vi "Dashboard Main.vi"() -> ()   [LabVIEW 2013]
uses:
  AnnieFramework/DoubleSolenoidAction.ctl
  AnnieFramework/CollectorAction.ctl
  AnnieFramework/CollectorWrapAction.ctl
  AnnieFramework/CatchAction.ctl
  AnnieFramework/AutoStates.ctl
  AnnieFramework/RollerAction.ctl
  AnnieFramework/AutoMode.ctl
  AnnieFramework/PassState.ctl
  AnnieFramework/HotGoalDetectType.ctl
  AnnieFramework/LowGoalState.ctl
  <vilib>/sound2/lvsound2.llb/Sound Data Format.ctl
  TabEnum.ctl
  <vilib>/sound2/lvsound2.llb/Sampling Mode.ctl
  <vilib>/event_ctls.llb/eventvkey.ctl
  <vilib>/Rock Robotics/WPI/Dashboard/WPI_DashboardLogging Global.vi
  <vilib>/Utility/config.llb/Write Key (String).vi
  <vilib>/Utility/config.llb/Write Key (I32).vi
  <vilib>/sound2/lvsound2.llb/Sound Input Read (DBL).vi
  KariFramework/CheckImageDistance.vi
  <vilib>/Utility/config.llb/NI_LVConfig.lvlib
  <vilib>/Analysis/NI_AALPro.lvlib
panel:
  in  "Enable Vision":bool=TRUE
  out "Image Message":string="Timeout in Camera Communications"
  in  "Rec Mode":enum32{"Stop", "Record", "Playback"}(radio)
  in  "Dashboard Tab":T1(tab)
  in  "DisableKinect":bool=TRUE
  out "Version":string
  in  "XBox":bool
  in  "DisableLCD":bool=TRUE
  out "GroundPassState":T2
  in  "DisableRollerOut":bool=TRUE
  out "FrontSonar":dbl
  out "AtPressure":bool
  out "CatchState":T3
  out "CollectorWrapState":T4
  out "CollectorState":T5
  out "CollectorMotor":dbl
  out "ClapperState":T6
  out "RollerPneuState":T6
  out "FiringCylinder2":bool
  out "FiringCylinder1":bool
  out "Kicker":bool
  out "AutoDistanceDone?":bool
  out "BackSonar":dbl
  out "BottomLS":bool
  out "TopLS":bool
  in  "MaxMotorChange":dbl=1.5
  out "Error":bool
  out "Right Motor":dbl
  out "Left Motor":dbl
  in  "Camera Settings":T7={"Frame Rate"=30, "Compression"=30, "Size"=1} {"Frame Rate" scale=1.0..30.0; "Size" items=["640x480", "320x240", "160x120"]}
  out "Mode":T8(ring)=enum.""
  out "Camera IP":string="0.0.0.11"
  in  "DB Camera Config":bool
  out "fps":dbl format="%#.1g"
  out "Mbps":dbl format="%#.1g"
  out "Mbps 2":bool
  out "Pressure":i32
  out "RollerMotorState":T9
  in  "DisableServo":bool=TRUE
  out "ElevatedPassState":T2
  out "Arcade":bool
  out "TankDriveTime":dbl
  out "SonicShifter":bool
  out "StraightDrive":bool
  out "HalfDrive":bool
  out "ReverseDrive":bool
  out "LowGoalDumpState":T10
  out "KinectTriggered?":bool
  out "ServoAngle":dbl
  out "WebcamMatched? Copy":bool
  out "PitchDetected Copy":bool
  in  "PreScumbagWait":i32
  out "CheckGoalTime":u32
  in  "StartShootTime":i32=5000
  in  "DriveBackTime":i32=1000
  in  "DriveBackSpeed":dbl=-1.0
  in  "EndInLowGear?":bool=TRUE
  out "DriveElapsedTime":u32
  in  "AccelBackward":dbl=0.1
  in  "AccelForward":dbl=0.1
  in  "StartInLowGear?":bool=TRUE
  out "ShootTime":u32
  in  "BallSettleWait":i32=130
  in  "PreCheckGoalWait":i32=260
  in  "Slowdown":dbl=36.0
  in  "Brake":dbl=12.0
  in  "DriveDistance":dbl=36.0
  in  "DriveMinTime":i32=2000
  in  "DriveTimeout":i32=4000
  out "WasHot?":bool
  out "DriveTimeOut":bool
  out "CheckGoalTimedOut?":bool
  out "ElapsedTime":u32
  out "StateTime":u32
  out "CurrentState":T11
  out "RaiseArmTimedOut":bool
  out "LowerArmTimedOut":bool
  out "IDMatched?":bool
  in  "AutoID":i32=3061
  in  "AutoMode":T12=enum."OneBallCollector"
  in  "HotGoalType":T13
  in  "ResetSound?":bool
  out "Frequency":T14(graph)={"df"=0.0, "df"=2.205, "Power Spectrum (V^2 rms)"=array[5000 elements]}
  out "RawData":waveform(dbl)[](graph)=[{"t0"=timestamp(3478468008.2170343 s since 1904-01-01), "dt"=4.5351473922902495e-05, "Y"=array[10000 elements]}, {"t0"=timestamp(3478468008.2170343 s since 1904-01-01), "dt"=4.5351473922902495e-05, "Y"=array[10000 elements]}]
  out "MaxValue":dbl=1.242701184627817e-06 format="%#.5f"
  in  "Average":dbl=1.0
  in  "Freq Bandwidth":dbl=500.0 format="%#_13g"
  in  "Start Freq":dbl=4000.0 format="%#_13g"
  in  "SoundFormat":T15={"sample rate (S/s)"=22050.0, "number of channels"=2, "bits per sample"=16}
  in  "StopSoundDetect":bool
  in  "SoundCutoff":dbl=10.0 format="%#_13g"
  out "PitchDetected":bool
  in  "% Cutoff":dbl=0.5
  out "NumHot":i32
  out "NumProcessed":i32
  in  "NumSamples":i32=5
  out "ProcessImage?":bool
  in  "Finished?":bool
  in  "Hot?":bool
  in  "Score cutoff":dbl=0.5
  in  "Color System":u16(ring)=2 items=["RGB", "HSL", "HSV", "HSI"]
  out "Distance (ft)":dbl
  in  "Color Components":T16={"Hue"={112.0, 144.0}, "Sat"={202.0, 255.0}, "Val"={237.0, 255.0}} {"Val" scale=0.0..255.0; "Sat" scale=0.0..255.0; "Hue" scale=0.0..255.0 scale format="%#_3g"}
  out "LoopTime":u32=500
  in  "Calibrate?":bool
  in  "Reset?":bool
  in  "SaveCameraImage?":bool=TRUE
  in  "TestWebcam?":bool
  in  "RunWebcam?":bool
  out "WebcamImagesProcessed":i32
  in  "ResetWebcam?":bool
  in  "WebcamImages":i32=1
  in  "SaveWebcamImage?":bool
  out "WebcamMatched?":bool
  in  "WebcamStartTime (ms)":i32=2000
  in  "StopWebcam?":bool
  out "WebcamImage":T17(plugin-control)
  in  "height":i32=480
  in  "width":i32=640
  in  "driver":i32
  in  "Test Slider":dbl(slide) scale=0.0..100.0 scale format="%#_3g"
  in  "On/Off":bool caption="Solenoid"
  in  "Test Name":u16(ring) items=["Select the test to run...", "Example Test", "-------------------------------", "List of tests is built in robot code.", "Replace with your own automated tests."]
  in  "Test Tree":string(tree)
  in  "Motor":cluster{"Value":dbl, "Enable":bool} {"Value" scale=-1.0..1.0 scale format="%#_3g"}
  out "Progress":T18 {"Test Progress" scale=0.0..100.0}
  in  "Rev/Fwd":cluster{"Forward":bool, "Reverse":bool}
  in  "Test Ring":u16(ring) items=["Auto", "Fixed indoor", "Fixed outdoor 1", "Fixed outdoor 2", "Fixed fluorescent 1", "Fixed fluorescent 2", "Hold current"]
  in  "Listbox":i32(listbox)
  out "Tree":string(tree)
  out "ClosePressure":bool
  out "CloseDist":bool
  out "FarDist":bool
  out "Timer":u32
  in  "CountdownStartTime":u32=10
  in  "AutoLength":u32=10
  in  "TeleopLength":u32=140
  out "Status":T19(ring)
  in  "Beep?":bool=TRUE
  out "SoundFilePath":path
  out "Errors":T20(array[cluster])
  in  "Reset":bool
  out "Camera Image":T17(plugin-control)
  # "DRIVE"
  # "GENERAL"
  # "OUTPUT"
  # "CONFIG"
  # "DEPRECATED"
  # "COUNTDOWN"
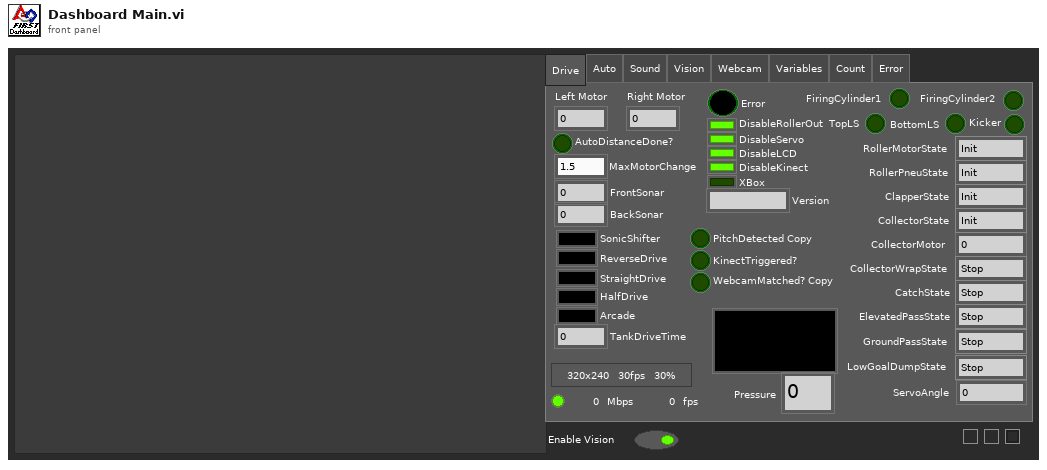
[diagram p1: front panel]
types:
  T1 = enum32{"Drive", "Auto", "Sound", "Vision", "Webcam", "Test", "Checklist", "Variables", "Count", "Error"}
  T2 = typedef "PassState.ctl" = enum16{"Stop", "Pass"}
  T3 = typedef "CatchAction.ctl" = enum16{"Stop", "PreCatch", "Catch"}
  T4 = typedef "CollectorWrapAction.ctl" = enum16{"Stop", "PreCollect", "Collect"}
  T5 = typedef "CollectorAction.ctl" = enum16{"Init", "Raise", "Lower", "Stop", "GetStatus"}
  T6 = typedef "DoubleSolenoidAction.ctl" = enum16{"Init", "Middle", "In", "Out"}
  T7 = cluster{"Frame Rate":i32, "Compression":i32, "Size":u16}
  T8 = enum8{"Tele-Op Disabled", "Tele-Op Enabled", "Auto Disabled", "Auto Enabled", "Test Disabled", "Test Enabled", ""}
  T9 = typedef "RollerAction.ctl" = enum16{"Init", "Off", "Forward", "Reverse"}
  T10 = typedef "LowGoalState.ctl" = enum16{"Stop", "Shoot"}
  T11 = typedef "AutoStates.ctl" = enum16{"Init", "LowerArmCheckGoal", "DriveBack", "Collect", "StopCollect", "LiftArm", "RaiseServo", "Drive", "ShootCollectorUp", "RaiseArm", "ShootCollectorDown", "Rotate1", "Rotate2", "Stop"}
  T12 = typedef "AutoMode.ctl" = enum16{"OneBallFront", "OneBallCollector", "TwoBallNormal", "TwoBallHot"}
  T13 = typedef "HotGoalDetectType.ctl" = enum16{"VisionTarget", "Kinect", "SoundDetect", "Webcam"}
  T14 = cluster{"df":dbl, "df":dbl, "Power Spectrum (V^2 rms)":dbl[]}
  T15 = typedef "Sound Data Format.ctl" = cluster{"sample rate (S/s)":dbl, "number of channels":i32, "bits per sample":i32}
  T16 = cluster{"Hue":cluster{dbl, dbl}, "Sat":cluster{dbl, dbl}, "Val":cluster{dbl, dbl}}
  T17 = typedef "IMAQ Image.ctl" = refnum<image>
  T18 = cluster{"Test Progress":u8, "Test Progress Text":string}
  T19 = enum8{"Disconnected", "E-Stop", "Disabled", "Enabled"}
  T20 = cluster{"status":bool, "code":i32, "location":string, "source":string}[]
  T21 = typedef "TabEnum.ctl" = enum32{"Drive", "Auto", "Sound", "Vision", "Webcam", "Variables", "Countdown", "Error"}
  T22 = typedef "Sampling Mode.ctl" = i32
  T23 = typedef "Image Type" = u32
  T24 = typedef "NI_LVConfig.lvlib/Config Data RefNum.ctl" = refnum<k1>
  T25 = typedef "Sound Input Task ID.ctl" = u32
  T26 = typedef "Sound Output Task ID.ctl" = u32
  T27 = cluster{"Digital Inputs":bool[], "Digital Outputs":bool[]}
  T28 = cluster{"Competition mode":bool, "Robot Link":bool, "Autonomous":bool, "Enabled":bool, "E-Stop":bool, "Simulated":bool, "TestMode":bool, "Docked Window":bool}
  T29 = typedef "CountdownAction.ctl" = enum16{"Start", "Reset", "Continue", "Idle"}
  T30 = cluster{"Boolean":bool, "Numeric":i32, "String":string, "String":string}[]
  T31 = cluster{cluster{dbl, dbl}, cluster{dbl, dbl}, cluster{dbl, dbl}}
  T32 = typedef "eventvkey.ctl" = enum16{"ASCII", "Enter", "Return", "Shift", "Ctrl", "Alt", "Cmd", "Opt", "Caps", "NumLock", "Clear", "Break", "Up", "Down", "Left", "Right", "Insert", "Delete", "Home", "End", "PageUp", "PageDown", "Escape", "Help", "Pause", "ScrollLock", "F1", "F2", "F3", "F4", "F5", "F6", "F7", "F8", "F9", "F10", "F11", "F12", "F13", "F14", "F15", "F16", "F17", "F18", "F19", "F20", "F21", "F22", "F23", "F24", "Play", "VolumeUp", "VolumeDown", "Mute", "Two Byte Char"}
  T33 = cluster{"Image Size":bool, "Image Type":bool, "Pixel Value":bool, "ROI Information":bool, "Zoom Factor":bool}
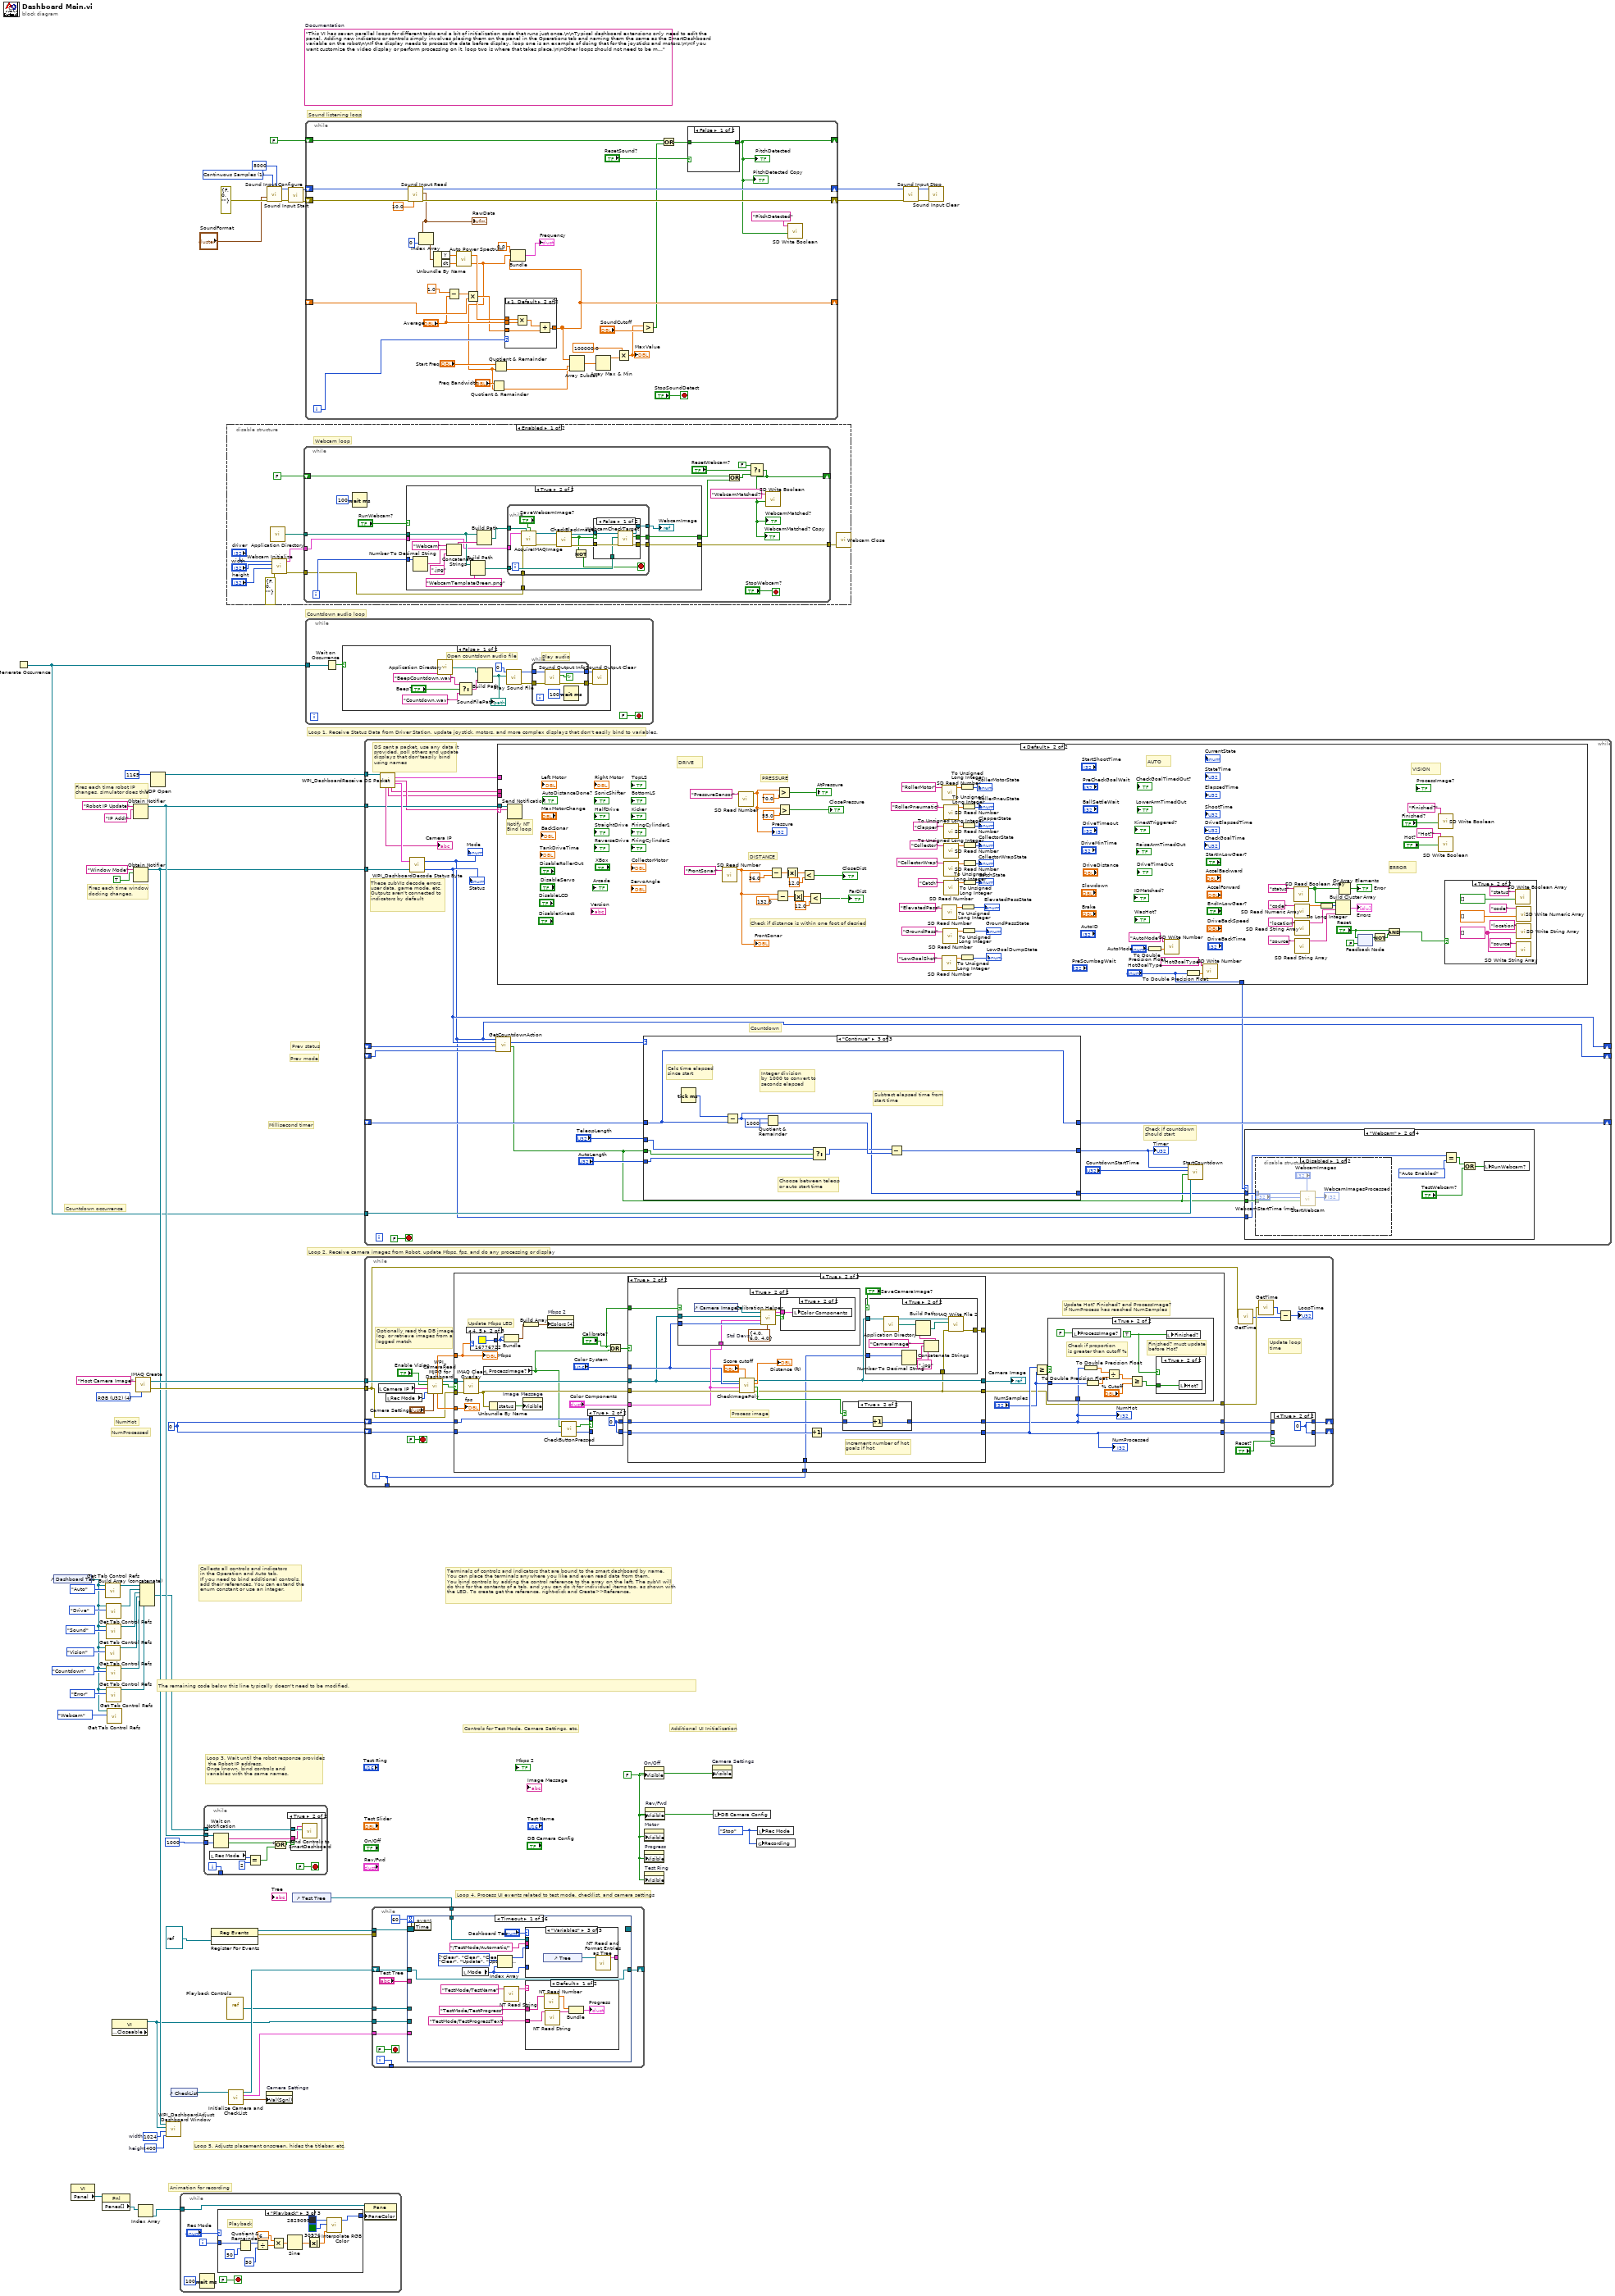
[diagram p0: block diagram]
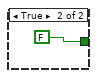
[diagram p2: hidden frame]
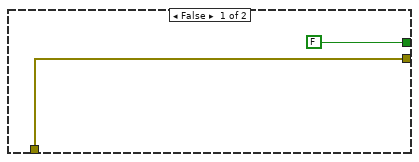
[diagram p4: hidden frame]
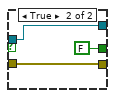
[diagram p5: hidden frame]
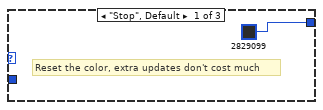
[diagram p8: hidden frame]
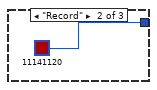
[diagram p9: hidden frame]
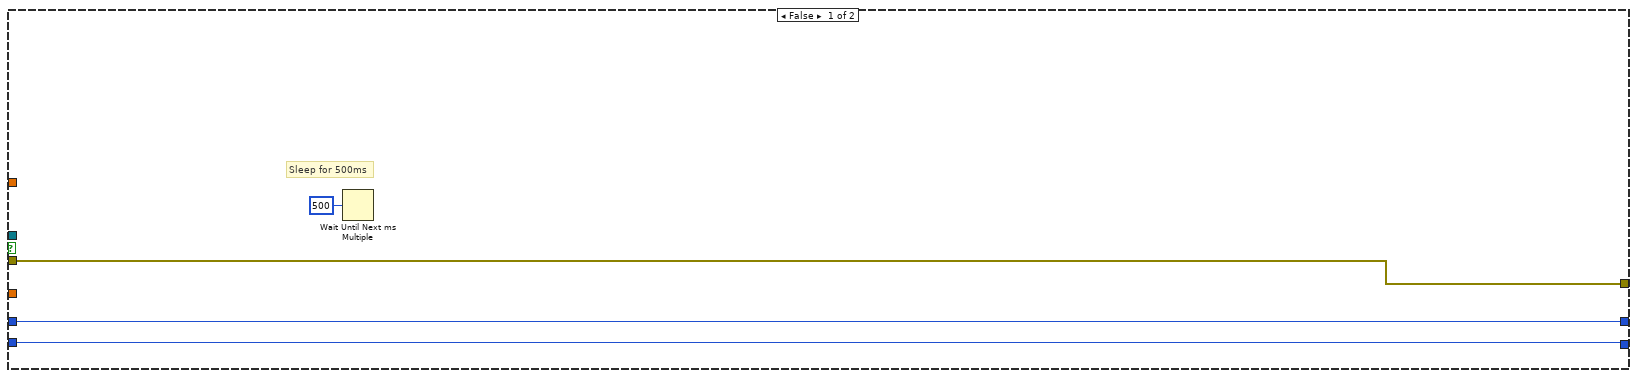
[diagram p12: hidden frame]
diagram:
  w23 = T22 1 items=["Finite Samples", "Continuous Samples"] ("sample mode")
  w26 = 0
  w32 = enum32{"Stop", "Record", "Playback"}."Stop" ("Rec Mode")
  w35 = 400  # height
  w36 = 1024  # width
  w49 = FALSE ("Visible")
  (unwired) "This VI has seven parallel loops for different tasks and a bit of initialization code that runs just once.\n\nTypical dashboard extensions only need to edit the panel. Adding new indicators or controls simply involves placing them on the panel in the Operations tab and naming them the same as the SmartDashboard variable on the robot\n\nIf the display needs to process the data before display, loop one is an example of doing that for the joysticks and motors.\n\nIf you want customize the video display or perform processing on it, loop two is where that takes place.\n\nOther loops should not need to be modified. They are pretty standard, and document the task they perform."  # Documentation
  w58 = T23 4 items=["Grayscale (U8)", "Grayscale (I16)", "Grayscale (SGL)", "Complex (CSG)", "RGB (U32)", "HSL (U32)", "RGB (U64)"] ("Image Type")
  # "Sound listening loop"
  # "Prev mode"
  # "Countdown audio loop"
  # "Countdown occurrence"
  # "Millisecond timer"
  # "Prev status"
  # "NumProcessed"
  # "NumHot"
  # "Controls for Test Mode, Camera Settings, etc."
  # "Additional UI Initialization"
  # "Animation for recording"
  # "Fires each time robot IP\nchanges, simulator does this"
  # "Fires each time window\ndocking changes."
  # "Collects all controls and indicators\nin the Operation and Auto tab.\nIf you need to bind additional controls,\nadd their references. You can extend the\nenum constant or use an integer."
  # "The remaining code below this line typically doesn't need to be modified."
  # "Loop 4. Process UI events related to test mode, checklist, and camera settings"
  # "Terminals of controls and indicators that are bound to the smart dashboard by name.\nYou can place the terminals anywhere you like and even read data from them.\nYou bind controls by adding the control reference to the array on the left. The subVI will\ndo this for the contents of a tab, and you can do it for individual items too, as shown with\nthe LED. To create get the reference, right-click and Create>>Reference."
  # "Loop 3. Wait until the robot response provides\n the Robot IP address.\nOnce known, bind controls and\nvariables with the same names."
  # "Loop 5. Adjusts placement onscreen, hides the titlebar, etc."
  # "Loop 1. Receive Status Data from Driver Station, update joystick, motors, and more complex displays that don't easily bind to variables."
  # "Loop 2. Receive camera images from Robot, update Mbps, fps, and do any processing or display"
  n1 = Generate Occurrence() -> (w25:refnum<k4>)
  n2 = control-ref of="Dashboard Tab"() -> (w2:refnum<vi>)
  n3 = property class="VI"() -> ("Panel"=w43:refnum<vi>)  [unwired: 2 in, 2 out]
  n4 = property class="Pnl"(reference=w43) -> ("Panes[]"=w44:refnum<vi>[])  [unwired: 1 in, 2 out]
  n5 = call <vilib>:"Get Tab Control Refs.vi"("Page Index"=TabEnum."Auto" ("Dashboard Tab"), "TabControl in"=w2) -> ("ControlsOnPage"=w30:refnum<vi>[])  [unwired: 9 in]
  n6 = call <vilib>:"Get Tab Control Refs.vi"("Page Index"=TabEnum."Vision" ("Dashboard Tab"), "TabControl in"=w2) -> ("ControlsOnPage"=w5:refnum<vi>[])  [unwired: 9 in]
  n7 = call <vilib>:"Get Tab Control Refs.vi"("Page Index"=TabEnum."Drive" ("Dashboard Tab"), "TabControl in"=w2) -> ("ControlsOnPage"=w27:refnum<vi>[])  [unwired: 9 in]
  n8 = call <vilib>:"Get Tab Control Refs.vi"("Page Index"=TabEnum."Sound" ("Dashboard Tab"), "TabControl in"=w2) -> ("ControlsOnPage"=w6:refnum<vi>[])  [unwired: 9 in]
  n9 = call <vilib>:"Get Tab Control Refs.vi"("Page Index"=TabEnum."Countdown" ("Dashboard Tab"), "TabControl in"=w2) -> ("ControlsOnPage"=w4:refnum<vi>[])  [unwired: 9 in]
  n10 = call <vilib>:"Get Tab Control Refs.vi"("Page Index"=TabEnum."Error" ("Dashboard Tab"), "TabControl in"=w2) -> ("ControlsOnPage"=w3:refnum<vi>[])  [unwired: 9 in]
  n11 = call <vilib>:"Get Tab Control Refs.vi"("Page Index"=TabEnum."Webcam" ("Dashboard Tab"), "TabControl in"=w2) -> ()  [unwired: 9 in, 1 out]
  n12 = property class="VI" props=["Front Panel.Closeable"]() -> (reference out=w31:refnum<vi>)  [unwired: 2 in, 2 out]
  n13 = Obtain Notifier(name (unnamed)="Robot IP Update", notification data type="IP Addr" ("name (unnamed)")) -> (notifier out=w52:refnum<notifier>)  [unwired: 2 in, 2 out]
  n14 = Obtain Notifier(name (unnamed)="Window Mode", notification data type=TRUE) -> (notifier out=w34:refnum<notifier>)  [unwired: 2 in, 2 out]
  n15 = call "IMAQ Create"("Image Name"="Host Camera Image", "Image Type"=w58) -> ("New Image"=w56:T17, "error out"=w55:errorcluster)  [unwired: 2 in, 1 out]
  n16 = Index Array(array=w44) -> (element=w42:refnum<vi>)  [unwired: 1 in]
  n17 = Build Array (concatenate)(w30, w27, w6, w5, w4, w3) -> (w29:refnum<vi>[])
  n18 = UDP Open(11:u16 1165 ("port")) -> (port=w59:refnum<k16>)  [unwired: 2 in, 4 out]
  n19 = call <vilib>:"WPI_DashboardAdjust Dashboard Window.vi"("height"=w35, "width"=w36, "reference in"=w31, "Notifier in"=w34) -> ()  [unwired: 8 in]
  n20 = control-ref of="CheckList"() -> (w33:refnum<vi>)
  n21 = while {
    tunnel: w42 -> [w62]
    i -> [w65]
    stop <- FALSE stop-if-true
    n22 = Wait (ms)(milliseconds to wait=u32 100) -> ()  [unwired: 1 out]
    n23 = case shown="\"Playback\"" "Rec Mode" {
      tunnel: w65 -> [_ _ w80]
      tunnel: [u32 2829099 ("Base Color") u32 11141120 ("Target Color") w69] -> w61
      frame "Stop", Default {
        # "Reset the color, extra updates don't cost much"
      }
      frame "Record" {
      }
      frame "Playback" {
        # "Playback"
        n24 = Quotient & Remainder(x=w80, y=u32 50 ("milliseconds to wait")) -> (x-y*floor(x/y)=w76:u32)  [unwired: 1 out]
        n25 = Divide(x=w76, y=u32 50 ("milliseconds to wait")) -> (x/y=w73:dbl)
        n26 = Multiply(x=6.283185307179586, y=w73) -> (x*y=w78:dbl)
        n27 = Sine(x=w78) -> (sin(x)=w77:dbl)
        n28 = Absolute Value(x=w77) -> (abs(x)=w70:dbl)
        n29 = call "Interpolate RGB Color.vi"("Proportion"=w70, "Target Color"=u32 30976, "Base Color"=u32 2829099) -> ("Result Color"=w69:u32)  [unwired: 8 in]
      }
    }
    n30 = property class="Pane"(reference=w62, "PaneColor"=w61) -> ()  [unwired: 1 in, 2 out]
  }
  n31 = while {
    tunnel: w29 -> [w91]
    tunnel: w52 -> [w89]
    tunnel: [w87] -> _
    tunnel: u32 1000 ("milliseconds to wait") -> [w86]
    i -> [w87]
    stop <- FALSE stop-if-true
    n32 = local read "Rec Mode"() -> (w82:enum32{"Stop", "Record", "Playback"})
    n33 = Wait on Notification(notifier=w89, timeout in ms (-1)=w86) -> (notification=w88:string, timed out?=w84:bool)  [unwired: 2 in, 2 out]
    n34 = Equal?(x=w82, y=u16 2 ("Rec Mode")) -> (x = y?=w83:bool)
    n35 = Compound Arithmetic op=OR(invert w84, w83) -> (w85:bool)
    n36 = case shown="True" w85 {
      tunnel: w91 -> [_ w93]
      tunnel: w88 -> [_ w92]
      frame False {
      }
      frame True {
        n37 = call <vilib>:"Bind Controls to SmartDashboard.vi"("Bound Control Refs"=w93, "Server IP Address"=w92) -> ()  [unwired: 10 in]
      }
    }
  }
  n38 = register-events(refnum<vi> refnum) -> (reference out=w40:refnum<event-registration>, error out=w39:errorcluster)  [unwired: 2 in]
  n39 = disable-structure shown="Enabled" {
    frame Enabled {
      # "Webcam loop"
      n40 = call <vilib>:"Application Directory.vi"() -> ("Application Directory"=w94:path)
      n41 = call "Webcam Initialize.vi"("error in"=errorcluster {"status"=FALSE, "code"=0, "source"=""}, "height (240)"="height", "width (320)"="width", "driver (0)"="driver") -> ("error out"=w97:errorcluster, "webcam image out"=w98:cluster{"image":u8[], "width":i32, "height":i32})  [unwired: 4 in, 1 out]
      n42 = while {
        tunnel: w94 -> [w117]
        tunnel: w98 -> [w115]
        tunnel: w97 -> [w114]
        tunnel: [w113] -> w96
        shift-right: [w103] -> _
        shift-left: FALSE -> [w109]
        i -> [w116]
        stop <- "StopWebcam?" stop-if-true
        n43 = Wait (ms)(milliseconds to wait=u32 100) -> ()  [unwired: 1 out]
        n44 = case shown="True" "RunWebcam?" {
          tunnel: [w118 w133] -> w113
          tunnel: [FALSE ("MatchFound?") w132] -> w108
          tunnel: w116 -> [_ w130]
          tunnel: w117 -> [_ w125]
          tunnel: w115 -> [_ w122]
          tunnel: w114 -> [w118 w121]
          frame False {
          }
          frame True {
            n45 = Number To Decimal String(number=w130) -> (decimal integer string=w129:string)  [unwired: 1 in]
            n46 = Concatenate Strings("Webcam", w129, ".jpg" ("string")) -> (w128:string)
            n47 = Build Path(base path=w125, name or relative path="WebcamTemplateGreen.png") -> (appended path=w124:path)
            n48 = Build Path(base path=w125, name or relative path=w128) -> (appended path=w127:path)
            n49 = while {
              tunnel: [w147] -> w133
              tunnel: [w146] -> w132
              tunnel: w127 -> [w145]
              tunnel: w124 -> [w143]
              tunnel: w122 -> [w136]
              tunnel: w121 -> [w135]
              tunnel: [w134] -> w120
              stop <- w137 stop-if-true
              n50 = call "AcquireIMAQImage.vi"("ImagePath"=w145, "SaveToDisk?"="SaveWebcamImage?", "error in"=w135, "webcam image in"=w136) -> ("error out"=w142:errorcluster, "ImageOut"=w140:T17)  [unwired: 6 in]
              n51 = call "CheckBlackImage.vi"("error in"=w142, "Image In"=w140) -> ("error out"=w141:errorcluster, "Black?"=w138:bool, "Image Out"=w139:T17)  [unwired: 7 in]
              n52 = Not(x=w138) -> (.not. x?=w137:bool)
              n53 = case shown="False" w138 {
                tunnel: w139 -> [w153 w154]
                tunnel: w141 -> [w152 w156]
                tunnel: [w151 w156] -> w147
                tunnel: [w150 FALSE ("MatchFound?")] -> w146
                tunnel: w143 -> [w149 _]
                tunnel: [w148 w154] -> w134
                frame False {
                  n54 = call "WebcamCheckTarget.vi"("error in"=w152, "TemplatePath"=w149, "ImageIn"=w153) -> ("error out"=w151:errorcluster, "MatchFound?"=w150:bool, "Image Out"=w148:T17)  [unwired: 6 in]
                }
                frame True {
                }
              }
            }
            "WebcamImage" <- w120
          }
        }
        n55 = Or(x=w109, y=w108) -> (x .or. y?=w106:bool)
        n56 = Select(t=FALSE, s="ResetWebcam?", f=w106) -> (s? t:f=w103:bool)
        "WebcamMatched?" <- w103
        "WebcamMatched? Copy" <- w103
        n57 = call <vilib>:"SD Write Boolean.vi"("Boolean"=w103, "Name"="WebcamMatched?") -> ()  [unwired: 8 in, 2 out]
      }
      n58 = call "Webcam Close.vi"("error in"=w96) -> ()  [unwired: 9 in, 1 out]
    }
    frame Disabled {
    }
  }
  n59 = vi-ref "Playback Controls.vi"() -> (w41:refnum<vi>)
  n60 = call "Initialize Camera and CheckList.vi"("ListBox in"=w33) -> ("Cluster"=w47:cluster{"value":i32, "value":i32, "index":i32}, "Array"=w48:cluster{string[]}[], "File Refnum"=w46:T24)  [unwired: 8 in]
  n61 = property on="Camera Settings" class="Clust (strict)"("Val(Sgnl)"=w47) -> ()  [unwired: 2 in, 2 out]
  n62 = call <vilib>:"Sound Input Configure.vi"("number of samples/ch"=8000, "sample mode"=w23, "error in (no error)"=errorcluster {"status"=FALSE, "code"=0, "source"=""}, "sound format"="SoundFormat") -> ("error out"=w20:errorcluster, "task ID"=w21:T25)  [unwired: 6 in]
  n63 = call <vilib>:"Sound Input Start.vi"("error in (no error)"=w20, "task ID"=w21) -> ("error out"=w19:errorcluster, "task ID out"=w18:T25)  [unwired: 8 in]
  n64 = control-ref of="Test Tree"() -> (w45:refnum<vi>)
  n65 = while {
    shift-right: [w189] -> w17
    shift-left: w19 -> [w191]
    shift-right: [w190] -> w16
    shift-left: w18 -> [w192]
    shift-right: [w186] -> _
    shift-left: _ -> [w188]
    shift-right: [w157] -> _
    shift-left: FALSE -> [w162]
    i -> [w187]
    stop <- "StopSoundDetect" stop-if-true
    n66 = call-poly <vilib>:"Sound Input Read.vi"("timeout (sec)"=10.0, "error in (no error)"=w191, "task ID"=w192) -> ("error out"=w189:errorcluster, "data"=w184:waveform(dbl)[], "task ID out"=w190:T25)  [unwired: 6 in]
    "RawData" <- w184
    n67 = Index Array(array=w184, index=0) -> (element=w180:waveform(dbl))
    n68 = Unbundle By Name(w180) -> ("Y"=w181:dbl[], "dt"=w178:dbl)
    n69 = Subtract(x=1.0, y="Average") -> (x-y=w174:dbl)
    n70 = call <vilib>:"Auto Power Spectrum.vi"("dt"=w178, "Signal (V)"=w181) -> ("df"=w170:dbl, "Power Spectrum (V^2 rms)"=w177:dbl[])
    n71 = Multiply(x=w174, y=w188) -> (x*y=w173:dbl[])
    n72 = Quotient & Remainder(x="Freq Bandwidth", y=w170) -> (floor(x/y)=w168:dbl)  [unwired: 1 out]
    n73 = Quotient & Remainder(x="Start Freq", y=w170) -> (floor(x/y)=w169:dbl)  [unwired: 1 out]
    n74 = case shown="1, Default" w187 {
      tunnel: w177 -> [w196 w201]
      tunnel: "Average" -> [_ w200]
      tunnel: w173 -> [_ w198]
      tunnel: [w196 w197] -> w186
      frame 0 {
      }
      frame 1, Default {
        n75 = Multiply(x=w201, y=w200) -> (x*y=w199:dbl[])
        n76 = Add(x=w199, y=w198) -> (x+y=w197:dbl[])
      }
    }
    n77 = Bundle("df"=0.0, "df"=w170, "Power Spectrum (V^2 rms)"=w186) -> (→"Frequency":T14)  [unwired: 1 in]
    n78 = Array Subset(array=w186, index=w169, length=w168) -> (w167:dbl[])
    n79 = Array Max & Min(array=w167) -> (max value=w166:dbl)  [unwired: 3 out]
    n80 = Multiply(x=100000.0, y=w166) -> (x*y=w163:dbl)
    "MaxValue" <- w163
    n81 = Greater?(x=w163, y="SoundCutoff") -> (0:w161:bool)
    n82 = Or(x=w162, y=w161) -> (x .or. y?=w160:bool)
    n83 = case shown="False" "ResetSound?" {
      tunnel: w160 -> [w194 _]
      tunnel: [w194 FALSE] -> w157
      frame False {
      }
      frame True {
      }
    }
    "PitchDetected" <- w157
    "PitchDetected Copy" <- w157
    n84 = call <vilib>:"SD Write Boolean.vi"("Boolean"=w157, "Name"="PitchDetected") -> ()  [unwired: 8 in, 2 out]
  }
  n85 = while {
    tunnel: w25 -> [w202]
    stop <- FALSE stop-if-true
    n86 = Wait on Occurrence(2:w202) -> (0:w204:bool)  [unwired: 2 in]
    n87 = case shown="False" w204 {
      frame False {
        # "Play audio"
        # "Open countdown audio file"
        n88 = call <vilib>:"Application Directory.vi"() -> ("Application Directory"=w205:path)
        n89 = Select(t="BeepCountdown.wav" ("name or relative path"), s="Beep?", f="Countdown.wav" ("name or relative path")) -> (s? t:f=w207:string)
        n90 = Build Path(base path=w205, name or relative path=w207) -> (appended path=w206:path)
        "SoundFilePath" <- w206
        n91 = call <vilib>:"Play Sound File.vi"("path"=w206, "device ID"=u32 0) -> ("error out"=w214:errorcluster, "task ID"=w213:T26)  [unwired: 8 in]
        n92 = while {
          tunnel: w214 -> [w216]
          tunnel: w213 -> [w220]
          tunnel: [w219] -> w212
          tunnel: [w217] -> w211
          stop <- w218 continue-if-true
          n93 = call <vilib>:"Sound Output Info.vi"("error in (no error)"=w216, "task ID"=w220) -> ("error out"=w217:errorcluster, "is playing?"=w218:bool, "task ID out"=w219:T26)  [unwired: 6 in, 1 out]
          n94 = Wait (ms)(milliseconds to wait=u32 100) -> ()  [unwired: 1 out]
        }
        n95 = call <vilib>:"Sound Output Clear.vi"("error in (no error)"=w211, "task ID"=w212) -> ()  [unwired: 9 in, 1 out]
      }
      frame True {
      }
    }
  }
  n96 = while {
    tunnel: w59 -> [w244]
    tunnel: w52 -> [w241]
    tunnel: w34 -> [w243]
    shift-right: [w236] -> _
    shift-left: _ -> [w235]
    shift-right: [w233] -> _
    shift-left: _ -> [w232]
    tunnel: w25 -> [w227]
    shift-right: [w222] -> _
    shift-left: _ -> [w224]
    stop <- FALSE stop-if-true
    # "Check if countdown\nshould start"
    # "Countdown"
    # "DS sent a packet. use any data it\nprovided, poll others and update\ndisplays that don'teasily bind\nusing names"
    # "These subVIs decode errors, user data, game mode, etc.\nOutputs aren't connected to indicators by default"
    n97 = call <vilib>:"WPI_DashboardReceive DS Packet.vi"("Recv Socket"=w244) -> ("Driver Station"=w237:T27, "Robot IP Address"=w240:string, "Status"=w245:T28, "Camera IP Address"=→"Camera IP":string, "Low Priority User Data"=w239:string, "High Priority User Data"=w238:string)  [unwired: 1 in, 8 out]
    n98 = call <vilib>:"WPI_DashboardDecode Status Byte.vi"("Window Mode Notifier"=w243, "Status"=w245) -> ("Status"=w236:T19, "Mode"=w222:T8)
    "Mode" <- w222
    "Status" <- w236
    n99 = call "GetCountdownAction.vi"("PrevMode"=w224, "PrevStatus"=w235, "CurrentStatus"=w236, "CurrentMode"=w222) -> ("Teleop?"=w225:bool, "Action"=w234:T29)  [unwired: 6 in]
    n100 = case shown="Default" w240 {
      selector: w240 -> [_ w349]
      tunnel: w241 -> [_ w350]
      tunnel: w239 -> [_ _]
      tunnel: w238 -> [_ _]
      tunnel: w237 -> [_ _]
      tunnel: [_ "HotGoalType"] -> w223
      frame "0.0.0.0" {
        # "DS not sending packets, or no robot exists yet.\nDon't poll the variables"
      }
      frame Default {
        # "Check if distance is within one foot of desried"
        # "ERROR"
        # "DISTANCE"
        # "PRESSURE"
        # "VISION"
        # "AUTO"
        # "DRIVE"
        # "Notify NT\nBind loop"
        n101 = Send Notification(notification=w349, notifier=w350) -> ()  [unwired: 1 in, 2 out]
        n102 = call <vilib>:"SD Read Number.vi"("Name"="FrontSonar") -> ("Numeric"=w300:dbl)  [unwired: 8 in, 2 out]
        "FrontSonar" <- w300
        n103 = call <vilib>:"SD Read Number.vi"("Name"="PressureSensor") -> ("Numeric"=w299:dbl)  [unwired: 8 in, 2 out]
        "Pressure" <- w299
        n104 = Subtract(x=w300, y=36.0) -> (x-y=w307:dbl)
        n105 = Subtract(x=w300, y=132.0) -> (x-y=w302:dbl)
        n106 = Greater?(x=w299, y=70.0) -> (0:→"AtPressure":bool)
        n107 = Greater?(x=w299, y=55.0) -> (0:→"ClosePressure":bool)
        n108 = Absolute Value(x=w307) -> (abs(x)=w306:dbl)
        n109 = Absolute Value(x=w302) -> (abs(x)=w303:dbl)
        n110 = Less?(x=w306, y=12.0) -> (x < y?=→"CloseDist":bool)
        n111 = Less?(x=w303, y=12.0) -> (x < y?=→"FarDist":bool)
        n112 = call <vilib>:"SD Read Number.vi"("Name"="LowGoalShot") -> ("Numeric"=w283:dbl)  [unwired: 8 in, 2 out]
        n113 = call <vilib>:"SD Read Number.vi"("Name"="RollerMotor") -> ("Numeric"=w297:dbl)  [unwired: 8 in, 2 out]
        n114 = call <vilib>:"SD Read Number.vi"("Name"="ElevatedPass") -> ("Numeric"=w291:dbl)  [unwired: 8 in, 2 out]
        n115 = call <vilib>:"SD Read Number.vi"("Name"="GroundPass") -> ("Numeric"=w290:dbl)  [unwired: 8 in, 2 out]
        n116 = call <vilib>:"SD Read Number.vi"("Name"="RollerPneumatic") -> ("Numeric"=w327:dbl)  [unwired: 8 in, 2 out]
        n117 = call <vilib>:"SD Read Number.vi"("Name"="Clapper") -> ("Numeric"=w325:dbl)  [unwired: 8 in, 2 out]
        n118 = call <vilib>:"SD Read Number.vi"("Name"="Collector") -> ("Numeric"=w322:dbl)  [unwired: 8 in, 2 out]
        n119 = call <vilib>:"SD Read Number.vi"("Name"="CollectorWrap") -> ("Numeric"=w319:dbl)  [unwired: 8 in, 2 out]
        n120 = call <vilib>:"SD Read Number.vi"("Name"="Catch") -> ("Numeric"=w316:dbl)  [unwired: 8 in, 2 out]
        n121 = To Unsigned Long Integer(number=w297) -> (unsigned 32bit integer=→"RollerMotorState":u32)
        n122 = To Unsigned Long Integer(number=w283) -> (unsigned 32bit integer=→"LowGoalDumpState":u32)
        n123 = To Unsigned Long Integer(number=w291) -> (unsigned 32bit integer=→"ElevatedPassState":u32)
        n124 = To Unsigned Long Integer(number=w327) -> (unsigned 32bit integer=→"RollerPneuState":u32)
        n125 = To Unsigned Long Integer(number=w325) -> (unsigned 32bit integer=→"ClapperState":u32)
        n126 = To Unsigned Long Integer(number=w290) -> (unsigned 32bit integer=→"GroundPassState":u32)
        n127 = To Unsigned Long Integer(number=w322) -> (unsigned 32bit integer=→"CollectorState":u32)
        n128 = To Unsigned Long Integer(number=w319) -> (unsigned 32bit integer=→"CollectorWrapState":u32)
        n129 = To Unsigned Long Integer(number=w316) -> (unsigned 32bit integer=→"CatchState":u32)
        n130 = To Double Precision Float(number="AutoMode") -> (double precision float=w293:dbl)
        n131 = call <vilib>:"SD Write Number.vi"("Numeric"=w293, "Name"="AutoMode") -> ()  [unwired: 8 in, 2 out]
        n132 = To Double Precision Float(number="HotGoalType") -> (double precision float=w286:dbl)
        n133 = call <vilib>:"SD Write Number.vi"("Numeric"=w286, "Name"="HotGoalType") -> ()  [unwired: 8 in, 2 out]
        n134 = call <vilib>:"SD Read Boolean Array.vi"("Name"="status") -> ("Boolean Array"=w338:bool[])  [unwired: 8 in, 2 out]
        n135 = call <vilib>:"SD Read Numeric Array.vi"("Name"="code") -> ("Numeric Array"=w337:dbl[])  [unwired: 8 in, 2 out]
        n136 = call <vilib>:"SD Read String Array.vi"("Name"="location") -> ("String Array"=w336:string[])  [unwired: 9 in, 1 out]
        n137 = call <vilib>:"SD Read String Array.vi"("Name"="source") -> ("String Array"=w335:string[])  [unwired: 9 in, 1 out]
        n138 = To Long Integer(number=w337) -> (32bit integer=w343:i32[])
        n139 = Build Cluster Array(w338, w343, w336, w335) -> (→"Errors":T30)
        n140 = Or Array Elements(Boolean array=w338) -> (logical OR=→"Error":bool)
        n141 = feedback #1(FALSE ("Reset")) -> (w346:bool)
        n142 = feedback-in #1("Reset") -> ()
        n143 = Not(x=w346) -> (.not. x?=w345:bool)
        n144 = And(x="Reset", y=w345) -> (x .and. y?=w344:bool)
        n145 = call <vilib>:"SD Write Boolean.vi"("Boolean"="Finished?", "Name"="Finished?") -> ()  [unwired: 8 in, 2 out]
        n146 = call <vilib>:"SD Write Boolean.vi"("Boolean"="Hot?", "Name"="Hot?") -> ()  [unwired: 8 in, 2 out]
        n147 = case shown="True" w344 {
          frame False {
          }
          frame True {
            w351 = string[] [] ("String Array")
            n148 = call <vilib>:"SD Write Boolean Array.vi"("Boolean Array"=bool[] [], "Name"="status") -> ()  [unwired: 8 in, 2 out]
            n149 = call <vilib>:"SD Write Numeric Array.vi"("Numeric Array"=dbl[] [], "Name"="code") -> ()  [unwired: 8 in, 2 out]
            n150 = call <vilib>:"SD Write String Array.vi"("String Array"=w351, "Name"="location") -> ()  [unwired: 8 in, 2 out]
            n151 = call <vilib>:"SD Write String Array.vi"("String Array"=w351, "Name"="source") -> ()  [unwired: 8 in, 2 out]
          }
        }
      }
    }
    n152 = case shown="\"Continue\"" w234 {
      tunnel: "TeleopLength" -> [w262 _ w275]
      tunnel: "AutoLength" -> [w261 _ w274]
      tunnel: [w265 w266 w273] -> w229
      tunnel: [w264 w267 w272] -> w233
      tunnel: w232 -> [_ w267 w272]
      tunnel: w225 -> [w263 _ w276]
      tunnel: [u32 0 ("millisecond timer value") w266 w268] -> w226
      frame "Start", Default {
        # "Choose between auto and teleop start times"
        n153 = Select(t=w262, s=w263, f=w261) -> (s? t:f=w265:u32)
        n154 = Tick Count (ms)() -> (millisecond timer value=w264:u32)
      }
      frame "Reset", "Idle" {
        w266 = u32 0 ("AutoStartTime")
      }
      frame "Continue" {
        # "Subtract elapsed time from\nstart time"
        # "Choose between teleop\nor auto start time"
        # "Integer division\nby 1000 to convert to\nseconds elapsed"
        # "Calc time elapsed\nsince start"
        n155 = Tick Count (ms)() -> (millisecond timer value=w269:u32)
        n156 = Subtract(x=w269, y=w272) -> (x-y=w268:u32)
        n157 = Quotient & Remainder(x=w268, y=u32 1000) -> (floor(x/y)=w271:u32)  [unwired: 1 out]
        n158 = Select(t=w275, s=w276, f=w274) -> (s? t:f=w270:u32)
        n159 = Subtract(x=w270, y=w271) -> (x-y=w273:u32)
      }
    }
    "Timer" <- w229
    n160 = call "StartCountdown.vi"("CountdownOccurrence"=w227, "Teleop?"=w225, "CountdownStartTime"="CountdownStartTime", "Time"=w229) -> ()  [unwired: 8 in]
    n161 = case shown="\"Webcam\"" w223 {
      tunnel: w226 -> [_ w253 _ _]
      tunnel: w225 -> [_ w252 _ _]
      tunnel: w222 -> [_ w251 _ _]
      frame "VisionTarget", Default {
      }
      frame "Webcam" {
        n162 = disable-structure shown="Disabled" {
          disable-tunnel: w253 -> [w259 _]
          disable-tunnel: w252 -> [w258 _]
          frame Disabled {
            n163 = call "StartWebcam.vi"("NumWebcamImages"="WebcamImages", "Teleop?"=w258, "WebcamStartTime (ms)"="WebcamStartTime (ms)", "ElapsedTime (ms)"=w259) -> ("WebcamImagesProcessed"=→"WebcamImagesProcessed":i32, "ResetWebcam?"=w255:bool)  [unwired: 6 in]
          }
          frame Enabled {
          }
        }
        n164 = Equal?(x=w251, y=T8."Auto Enabled") -> (x = y?=w249:bool)
        n165 = Or(x=w249, y="TestWebcam?") -> (x .or. y?=w247:bool)
        n166 = local write "RunWebcam?"(w247) -> ()
      }
      frame "Kinect" {
      }
      frame "SoundDetect" {
      }
    }
  }
  n167 = while {
    tunnel: w56 -> [w379]
    tunnel: w55 -> [w364]
    tunnel: [w358] -> _
    shift-right: [w359] -> _
    shift-left: w26 -> [w369]
    shift-right: [w360] -> _
    shift-left: w26 -> [w370]
    i -> [w358]
    stop <- FALSE stop-if-true
    # "Update loop\ntime"
    # "Optionally read the DB image,\nlog, or retrieve images from a\nlogged match"
    n168 = local read "Camera IP"() -> (w372:string)
    n169 = local read "Rec Mode"() -> (w371:enum32{"Stop", "Record", "Playback"})
    n170 = call <vilib>:"WPI_CameraRead MJPG for Dashboard.vi"("Camera Settings"="Camera Settings", "Rec Mode"=w371, "Camera IP"=w372, "Enable"="Enable Vision", "Refnum in"=w379) -> ("Active"=w376:bool, "Refnum out"=w378:T17, "FPS"=w375:dbl, "Bandwidth (Mbps)"=w374:dbl)  [unwired: 3 in]
    n171 = case shown="True" w376 {
      tunnel: w378 -> [_ w410]
      tunnel: w374 -> [_ w409]
      tunnel: w375 -> [_ w408]
      tunnel: w370 -> [w385 w398]
      tunnel: w369 -> [w386 w397]
      tunnel: [w386 w403] -> w362
      tunnel: [w385 w402] -> w361
      tunnel: [w384 w400] -> w367
      tunnel: w364 -> [w384 w399]
      tunnel: w358 -> [_ w388]
      frame False {
        # "Sleep for 500ms"
        n172 = Wait Until Next ms Multiple(millisecond multiple=u32 500) -> ()  [unwired: 1 out]
      }
      frame True {
        # "Update Hot? Finished? and ProcessImage?\nIf NumProcess has reached NumSamples"
        # "Update Mbps LED"
        n173 = call "IMAQ Clear Overlay"("error in (no error)"=w399, "Image"=w410) -> ("error out"=w405:errorcluster, "Image Out"=w407:T17)  [unwired: 1 in, 7 out]
        n174 = case shown="4, 5" w409 {
          tunnel: [u32 6618880 ("Color Box") u32 16776722 ("Color Box") u32 16716800 ("Color Box")] -> w411
          frame Default {
          }
          frame 4, 5 {
          }
          frame 6.. {
          }
        }
        n175 = local read "ProcessImage?"() -> (w390:bool)
        n176 = Unbundle By Name(w405) -> ("status"=w414:bool)
        n177 = Bundle("Color Box"=w411, "Color Box"=w411) -> (w413:cluster{"Color Box":u32, "Color Box":u32})  [unwired: 1 out]
        n178 = property on="Image Message" class="Str"("Visible"=w414) -> ()  [unwired: 2 in, 2 out]
        n179 = Build Array(w413) -> (w412:cluster{"Color Box":u32, "Color Box":u32}[])
        n180 = property on="Mbps 2" class="Bool (strict)"("Colors [4]"=w412) -> ()  [unwired: 2 in, 2 out]
        n181 = call "CheckButtonPressed.vi"("Button"=w390) -> ("Pressed?"=w394:bool)  [unwired: 9 in, 1 out]
        n182 = case shown="True" w394 {
          tunnel: w398 -> [w416 _]
          tunnel: w397 -> [w415 _]
          tunnel: [w416 w417] -> w396
          tunnel: [w415 w417] -> w395
          frame False {
          }
          frame True {
            w417 = 0
          }
        }
        n183 = Or(x="Calibrate?", y=w390) -> (x .or. y?=w391:bool)
        n184 = case shown="True" w391 {
          tunnel: w407 -> [w428 w438]
          tunnel: [w428 w435] -> w406
          tunnel: w396 -> [w430 w444]
          tunnel: w395 -> [w431 w446]
          tunnel: w405 -> [w429 w447]
          tunnel: [w429 w434] -> w400
          tunnel: [w431 w445] -> w403
          tunnel: [w430 w443] -> w402
          tunnel: "Color Components" -> [_ w440]
          tunnel: "Color System" -> [_ w439]
          tunnel: "Calibrate?" -> [_ w437]
          tunnel: [_ w433] -> _
          tunnel: w388 -> [_ w432]
          frame False {
          }
          frame True {
            # "Process image"
            # "Increment number of hot\ngoals if hot"
            n185 = case shown="True" w437 {
              tunnel: w439 -> [_ w464]
              tunnel: w440 -> [_ w463]
              tunnel: w438 -> [_ w462]
              frame False {
              }
              frame True {
                w465 = cluster{"Hue":dbl, "Sat":dbl, "Val":dbl} {"Hue"=4.0, "Sat"=6.0, "Val"=4.0}  # Std Devs
                n186 = control-ref of="Camera Image"() -> (w461:refnum<vi>)
                n187 = call "Calibration Helper.vi"("Std Devs"=w465, "Color Mode"=w464, "Color Components"=w463, "Image"=w462, "Image Ctl Refnum"=w461) -> ("Changed"=w459:bool, "output color"=w460:T31)  [unwired: 5 in]
                n188 = case shown="True" w459 {
                  tunnel: w460 -> [_ w466]
                  frame False {
                  }
                  frame True {
                    n189 = local write "Color Components"(w466) -> ()
                  }
                }
              }
            }
            n190 = call-poly "CheckImagePoly.vi"("Score cutoff"="Score cutoff", "error in"=w447, "Color Components"=w440, "Color System"=w439, "Image"=w438) -> ("error out"=w434:errorcluster, "Hot?"=w441:bool, "Distance (ft)"=→"Distance (ft)":dbl, "Image out"=w435:T17)  [unwired: 3 in]
            n191 = Increment(x=w446) -> (x+1=w445:i32)
            n192 = case shown="True" w441 {
              tunnel: w444 -> [w467 w469]
              tunnel: [w467 w468] -> w443
              frame False {
              }
              frame True {
                n193 = Increment(x=w469) -> (x+1=w468:i32)
              }
            }
            n194 = case shown="True" "SaveCameraImage?" {
              tunnel: w435 -> [_ w458]
              tunnel: w434 -> [_ w457]
              tunnel: [_ w456] -> w433
              tunnel: w432 -> [_ w453]
              frame False {
              }
              frame True {
                n195 = call <vilib>:"Application Directory.vi"() -> ("Application Directory"=w449:path)
                n196 = Number To Decimal String(number=w453) -> (decimal integer string=w452:string)  [unwired: 1 in]
                n197 = Concatenate Strings("CameraImage", w452, ".jpg" ("string")) -> (w450:string)
                n198 = Build Path(base path=w449, name or relative path=w450) -> (appended path=w455:path)
                n199 = call-poly "IMAQ Write File 2"("error in (no error)"=w457, "File Path"=w455, "Image"=w458) -> ("error out"=w456:errorcluster)  [unwired: 7 in, 1 out]
              }
            }
          }
        }
        "Camera Image" <- w406
        "NumHot" <- w402
        "NumProcessed" <- w403
        n200 = Greater Or Equal?(x=w403, y="NumSamples") -> (x >= y?=w404:bool)
        n201 = case shown="True" w404 {
          tunnel: w402 -> [_ w425]
          tunnel: "NumSamples" -> [_ w426]
          frame False {
          }
          frame True {
            w418 = TRUE ("Finished?")
            # "Finished? must update\nbefore Hot?"
            # "Check if proportion\nis greater than cutoff %"
            n202 = local write "ProcessImage?"(FALSE ("ProcessImage?")) -> ()
            n203 = To Double Precision Float(number=w425) -> (double precision float=w423:dbl)
            n204 = To Double Precision Float(number=w426) -> (double precision float=w424:dbl)
            n205 = Divide(x=w423, y=w424) -> (x/y=w422:dbl)
            n206 = Greater Or Equal?(x=w422, y="% Cutoff") -> (x >= y?=w420:bool)
            n207 = case shown="True" w418 {
              tunnel: w420 -> [_ w427]
              frame False {
              }
              frame True {
                n208 = local write "Hot?"(w427) -> ()
              }
            }
            n209 = local write "Finished?"(w418) -> ()
          }
        }
        "Mbps" <- w409
        "fps" <- w408
      }
    }
    n210 = call "GetTime.vi"("error in"=w364) -> ("Time"=w366:u32)
    n211 = call "GetTime.vi"("error in"=w367) -> ("Time"=w368:u32)
    n212 = case shown="True" "Reset?" {
      tunnel: w362 -> [w381 _]
      tunnel: w361 -> [w382 _]
      tunnel: [w382 w383] -> w360
      tunnel: [w381 w383] -> w359
      frame False {
      }
      frame True {
        w383 = 0
      }
    }
    n213 = Subtract(x=w368, y=w366) -> (x-y=→"LoopTime":u32)
  }
  n214 = while {
    tunnel: w48 -> [w480]
    shift-right: [w479] -> _
    shift-left: w46 -> [w478]
    tunnel: [w477] -> _
    tunnel: w45 -> [w476]
    tunnel: w41 -> [w475]
    tunnel: w40 -> [w474]
    tunnel: w39 -> [_]
    tunnel: w31 -> [w473]
    i -> [w477]
    stop <- FALSE stop-if-true
    n215 = event shown="[0] Timeout" {
      selector: w474 -> [_ _ _ _ _ _ _ _ _ _ _ _ _ _ _ _]
      dyn-events: [_ _ _ _ _ _ _ _ _ _ _ _ _ w718 _ _] -> _
      timeout: u32 60 ("milliseconds to wait") -> [_ _ _ _ _ _ _ _ _ _ _ _ _ _ _ _]
      tunnel: w476 -> [w490 _ _ _ _ _ _ _ _ _ _ _ _ _ _ _]
      tunnel: "Test Tree" -> [_ _ _ _ _ _ _ _ w687 w695 w697 w701 w709 _ _ _]
      tunnel: w480 -> [_ w514 _ _ _ _ w651 w681 _ _ _ _ _ _ _ _]
      tunnel: [w484 w513 w612 w617 w625 w637 w650 w674 w686 w693 w696 w700 w708 w720 w734 w735] -> w479
      tunnel: w478 -> [w484 w513 w612 w617 w625 w637 w649 w674 w686 w693 w696 w700 w708 w720 w734 w735]
      tunnel: w475 -> [_ _ _ _ _ _ _ _ _ _ _ _ _ w721 _ w738]
      tunnel: w473 -> [_ _ _ _ _ _ _ _ _ _ _ _ _ w716 _ _]
      event Timeout {
        w489 = enum16{"Update", "Clear"}[] [enum."Clear", enum."Clear", enum."Clear", enum."Clear", enum."Update", enum."Update", enum."Clear"] items=["Update", "Clear"]
        n216 = event-data() -> ()  [unwired: 1 in, 1 out]
        n217 = local read "Mode"() -> (w487:T8)
        n218 = Index Array(array=w489, index=w487) -> (element=w488:enum16{"Update", "Clear"})
        n219 = call <vilib>:"NT Read String.vi"("Name"="TestMode/TestName") -> ("String"=w493:string)  [unwired: 9 in, 1 out]
        n220 = case shown="\"Variables\"" "Dashboard Tab" {
          tunnel: w490 -> [_ w503 _]
          tunnel: "/TestMode/Automatic/" ("Name Pattern") -> [_ w502 _]
          tunnel: w488 -> [_ w501 _]
          tunnel: w487 -> [_ w499 _]
          tunnel: [_ _ w505] -> _
          frame "Auto", Default {
          }
          frame "Test" {
            w498 = -2 ("Active Item:Row Number")
            n221 = call <vilib>:"NT Read and Format Entries as Tree.vi"("Operation"=w501, "Name Pattern"=w502, "Tree Refnum"=w503) -> ()  [unwired: 7 in, 2 out]
            n222 = Index Array(array=u32[] [14013909, 14013909, 14013909, 14013909, 14013909, 16777215, 14013909], index=w499) -> (element=w497:u32)
            n223 = property on="Test Tree" class="Tree (strict)"("Active Item Row Number"=w498, "ActiveColNum"=w498, "CellBG"=w497, "Active Item Row Number"=-1 ("Active Item:Row Number"), "CellBG"=u32 5789784 ("Color Box")) -> ()  [unwired: 2 in, 2 out]
          }
          frame "Variables" {
            n224 = control-ref of="Tree"() -> (w504:refnum<vi>)
            n225 = call <vilib>:"NT Read and Format Entries as Tree.vi"("Tree Refnum"=w504) -> ("Formatted Strings"=w505:cluster{"Name":string, "Value":string}[])  [unwired: 9 in, 1 out]
          }
        }
        n226 = case shown="Default" w493 {
          tunnel: "TestMode/TestProgress" ("Name") -> [w507 _]
          tunnel: "TestMode/TestProgressText" ("Name") -> [w506 _]
          frame Default {
            n227 = call <vilib>:"NT Read Number.vi"("Name"=w507) -> ("Numeric"=w508:dbl)  [unwired: 9 in, 1 out]
            n228 = call <vilib>:"NT Read String.vi"("Name"=w506) -> ("String"=w509:string)  [unwired: 9 in, 1 out]
            n229 = Bundle("Numeric"=w508, "String"=w509) -> (→"Progress":cluster{"Numeric":dbl, "String":string})  [unwired: 1 in]
          }
          frame "" {
            n230 = property on="Progress" class="Clust (strict)"("Visible"=FALSE) -> ()  [unwired: 2 in, 2 out]
            n231 = local write "Test Name"(u16 0) -> ()
          }
        }
      }
      event "Test Tree": Value Change {
        # "Show appropriate\ncontrols"
        n232 = event-data() -> ("CtlRef"=w517:refnum<vi>, "NewVal"=w515:string)  [unwired: 1 in]
        n233 = call <vilib>:"WPI_UtilitiesGetTreeIOName.vi"("NewVal"=w515, "TreeControl in"=w517) -> ("I/O Name"=w518:string)  [unwired: 9 in]
        n234 = case shown="\"Camera\"" w518 {
          selector: w518 -> [_ w525 _ w543 w552 _]
          tunnel: w515 -> [_ _ w540 w542 _ w559]
          tunnel: w514 -> [_ _ _ _ _ w558]
          frame Default {
            w520 = FALSE ("Visible")
            w519 = FALSE ("Visible")
            n235 = property on="Motor" class="Clust (strict)"("Visible"=w519) -> ()  [unwired: 2 in, 2 out]
            n236 = property on="Test Ring" class="Ring (strict)"("Visible"=w519) -> ()  [unwired: 2 in, 2 out]
            n237 = property on="Rev/Fwd" class="Clust (strict)"("Visible"=w520) -> ()  [unwired: 2 in, 2 out]
            n238 = property on="On/Off" class="Bool (strict)"("Visible"=w520) -> ()  [unwired: 2 in, 2 out]
            n239 = property on="Test Slider" class="Slide (strict)"("Visible"=w520) -> ()  [unwired: 2 in, 2 out]
          }
          frame "Motor", "PWM" {
            w526 = FALSE ("Visible")
            n240 = case shown="\"Motor\", Default" w525 {
              tunnel: [1.0 ("Value") -1.0 ("Value")] -> w524
              tunnel: [255.0 ("Value") 1.0 ("Value")] -> w523
              tunnel: [128.0 ("Value") 0.0 ("Value")] -> w522
              tunnel: [64.0 ("Value") 0.5 ("Value")] -> w521
              frame "PWM" {
              }
              frame "Motor", Default {
              }
            }
            n241 = property on="Motor" class="Clust (strict)"("Visible"=TRUE) -> ()  [unwired: 2 in, 2 out]
            n242 = property on="Value" class="Slide (strict)"("Value"=w522, "Scale.Minimum"=w524, "Scale.Maximum"=w523, "Scale.Increment"=w521) -> ()  [unwired: 2 in, 2 out]
            n243 = property on="On/Off" class="Bool (strict)"("Visible"=w526) -> ()  [unwired: 2 in, 2 out]
            n244 = property on="Test Slider" class="Slide (strict)"("Visible"=w526) -> ()  [unwired: 2 in, 2 out]
            n245 = property on="Test Ring" class="Ring (strict)"("Visible"=w526) -> ()  [unwired: 2 in, 2 out]
            n246 = property on="Rev/Fwd" class="Clust (strict)"("Visible"=w526) -> ()  [unwired: 2 in, 2 out]
          }
          frame "Servo" {
            w538 = FALSE ("Visible")
            n247 = call <vilib>:"NT Read Number.vi"("Name"=w540) -> ("Numeric"=w539:dbl)  [unwired: 9 in, 1 out]
            n248 = property on="Test Slider" class="Slide (strict)"("Visible"=TRUE, "Scale.Maximum"=170.0 ("Scale.Range:Maximum")) -> ()  [unwired: 2 in, 2 out]
            n249 = local write "Test Slider"(w539) -> ()
            n250 = property on="Motor" class="Clust (strict)"("Visible"=w538) -> ()  [unwired: 2 in, 2 out]
            n251 = property on="Rev/Fwd" class="Clust (strict)"("Visible"=w538) -> ()  [unwired: 2 in, 2 out]
            n252 = property on="On/Off" class="Bool (strict)"("Visible"=w538) -> ()  [unwired: 2 in, 2 out]
            n253 = property on="Test Ring" class="Ring (strict)"("Visible"=w538) -> ()  [unwired: 2 in, 2 out]
          }
          frame "Relay", "Solenoid" {
            w541 = FALSE ("Visible")
            n254 = property on="Motor" class="Clust (strict)"("Visible"=w541) -> ()  [unwired: 2 in, 2 out]
            n255 = property on="Test Slider" class="Slide (strict)"("Visible"=w541) -> ()  [unwired: 2 in, 2 out]
            n256 = Search and Replace String(input string=w542, search string="/Value  **", replace string="/Direction") -> (result string=w548:string)  [unwired: 5 in, 3 out]
            n257 = property on="Test Ring" class="Ring (strict)"("Visible"=w541) -> ()  [unwired: 2 in, 2 out]
            n258 = call <vilib>:"NT Read String.vi"("Name"=w548) -> ("String"=w546:string)  [unwired: 9 in, 1 out]
            n259 = Equal?(x="Both directions", y=w546) -> (x = y?=w544:bool)
            n260 = Not(x=w544) -> (.not. x?=w545:bool)
            n261 = property on="Rev/Fwd" class="Clust (strict)"("Visible"=w544) -> ()  [unwired: 2 in, 2 out]
            n262 = property on="On/Off" class="Bool (strict)"("Visible"=w545, "Caption.Text"=w543) -> ()  [unwired: 2 in, 2 out]
          }
          frame "Compressor", "Digital Out" {
            w551 = FALSE ("Visible")
            # "Get direction and finish"
            n263 = property on="Motor" class="Clust (strict)"("Visible"=w551) -> ()  [unwired: 2 in, 2 out]
            n264 = property on="Test Slider" class="Slide (strict)"("Visible"=w551) -> ()  [unwired: 2 in, 2 out]
            n265 = property on="Test Ring" class="Ring (strict)"("Visible"=w551) -> ()  [unwired: 2 in, 2 out]
            n266 = property on="On/Off" class="Bool (strict)"("Visible"=TRUE, "Caption.Text"=w552) -> ()  [unwired: 2 in, 2 out]
            n267 = property on="Rev/Fwd" class="Clust (strict)"("Visible"=FALSE) -> ()  [unwired: 2 in, 2 out]
          }
          frame "Camera" {
            n268 = call <vilib>:"Get Last Path Segment.vi"("String in"=w559) -> ("String out"=w560:string)  [unwired: 10 in]
            n269 = property on="On/Off" class="Bool (strict)"("Visible"=FALSE) -> ()  [unwired: 2 in, 2 out]
            n270 = property on="Motor" class="Clust (strict)"("Visible"=FALSE) -> ()  [unwired: 2 in, 2 out]
            n271 = property on="Rev/Fwd" class="Clust (strict)"("Visible"=FALSE) -> ()  [unwired: 2 in, 2 out]
            n272 = case shown="\"White Balance  **\"" w560 {
              tunnel: w559 -> [w566 w575 w584 w593 w602 _ w608]
              tunnel: w558 -> [w564 w572 w581 w590 w599 _ _]
              frame "Size  **" {
                n273 = Index Array(array=w564) -> (element=w563:cluster{string[]})  [unwired: 1 in]
                n274 = call <vilib>:"NT Read String.vi"("Name"=w566) -> ("String"=w565:string)  [unwired: 9 in, 1 out]
                n275 = Unbundle(w563) -> (w561:string[])
                n276 = Match First String(2:w561, 3:w565) -> (0:w562:i32)  [unwired: 1 out]
                n277 = property on="Test Ring" class="Ring (strict)"("Value"=w562, "Strings []"=w561) -> ()  [unwired: 2 in, 2 out]
                n278 = property on="Test Ring" class="Ring (strict)"("Visible"=TRUE) -> ()  [unwired: 2 in, 2 out]
                n279 = property on="Test Slider" class="Slide (strict)"("Visible"=FALSE) -> ()  [unwired: 2 in, 2 out]
              }
              frame "White Balance  **" {
                n280 = Index Array(array=w572, index=1) -> (element=w573:cluster{string[]})
                n281 = call <vilib>:"NT Read String.vi"("Name"=w575) -> ("String"=w574:string)  [unwired: 9 in, 1 out]
                n282 = Unbundle(w573) -> (w570:string[])
                n283 = Match First String(2:w570, 3:w574) -> (0:w569:i32)  [unwired: 1 out]
                n284 = property on="Test Ring" class="Ring (strict)"("Value"=w569, "Strings []"=w570) -> ()  [unwired: 2 in, 2 out]
                n285 = property on="Test Ring" class="Ring (strict)"("Visible"=TRUE) -> ()  [unwired: 2 in, 2 out]
                n286 = property on="Test Slider" class="Slide (strict)"("Visible"=FALSE) -> ()  [unwired: 2 in, 2 out]
              }
              frame "Exposure  **" {
                n287 = Index Array(array=w581, index=2) -> (element=w582:cluster{string[]})
                n288 = call <vilib>:"NT Read String.vi"("Name"=w584) -> ("String"=w583:string)  [unwired: 9 in, 1 out]
                n289 = Unbundle(w582) -> (w578:string[])
                n290 = Match First String(2:w578, 3:w583) -> (0:w579:i32)  [unwired: 1 out]
                n291 = property on="Test Ring" class="Ring (strict)"("Value"=w579, "Strings []"=w578) -> ()  [unwired: 2 in, 2 out]
                n292 = property on="Test Ring" class="Ring (strict)"("Visible"=TRUE) -> ()  [unwired: 2 in, 2 out]
                n293 = property on="Test Slider" class="Slide (strict)"("Visible"=FALSE) -> ()  [unwired: 2 in, 2 out]
              }
              frame "Exposure Priority  **" {
                n294 = Index Array(array=w590, index=3) -> (element=w591:cluster{string[]})
                n295 = call <vilib>:"NT Read String.vi"("Name"=w593) -> ("String"=w592:string)  [unwired: 9 in, 1 out]
                n296 = Unbundle(w591) -> (w587:string[])
                n297 = Match First String(2:w587, 3:w592) -> (0:w588:i32)  [unwired: 1 out]
                n298 = property on="Test Ring" class="Ring (strict)"("Value"=w588, "Strings []"=w587) -> ()  [unwired: 2 in, 2 out]
                n299 = property on="Test Ring" class="Ring (strict)"("Visible"=TRUE) -> ()  [unwired: 2 in, 2 out]
                n300 = property on="Test Slider" class="Slide (strict)"("Visible"=FALSE) -> ()  [unwired: 2 in, 2 out]
              }
              frame "Color Enable  **" {
                n301 = Index Array(array=w599, index=4) -> (element=w600:cluster{string[]})
                n302 = call <vilib>:"NT Read String.vi"("Name"=w602) -> ("String"=w601:string)  [unwired: 9 in, 1 out]
                n303 = Unbundle(w600) -> (w596:string[])
                n304 = Match First String(2:w596, 3:w601) -> (0:w597:i32)  [unwired: 1 out]
                n305 = property on="Test Ring" class="Ring (strict)"("Value"=w597, "Strings []"=w596) -> ()  [unwired: 2 in, 2 out]
                n306 = property on="Test Ring" class="Ring (strict)"("Visible"=TRUE) -> ()  [unwired: 2 in, 2 out]
                n307 = property on="Test Slider" class="Slide (strict)"("Visible"=FALSE) -> ()  [unwired: 2 in, 2 out]
              }
              frame Default {
                n308 = property on="Test Ring" class="Ring (strict)"("Visible"=FALSE) -> ()  [unwired: 2 in, 2 out]
                n309 = property on="Test Slider" class="Slide (strict)"("Visible"=FALSE) -> ()  [unwired: 2 in, 2 out]
              }
              frame "Brightness  **", "Color Level  **", "Compression  **", "FPS  **", "Sharpness  **" {
                n310 = call <vilib>:"NT Read Number.vi"("Name"=w608) -> ("Numeric"=w607:dbl)  [unwired: 9 in, 1 out]
                n311 = local write "Test Slider"(w607) -> ()
                n312 = property on="Test Slider" class="Slide (strict)"("Visible"=TRUE, "Scale.Maximum"=100.0 ("Scale.Range:Maximum")) -> ()  [unwired: 2 in, 2 out]
                n313 = property on="Test Ring" class="Ring (strict)"("Visible"=FALSE) -> ()  [unwired: 2 in, 2 out]
              }
            }
          }
        }
        n314 = property on="Progress" class="Clust (strict)"("Visible"=FALSE) -> ()  [unwired: 2 in, 2 out]
      }
      event "Test Name": Mouse Enter {
        # "Populate the ring with the list of tests"
        n315 = event-data() -> ()  [unwired: 1 in, 1 out]
        n316 = call <vilib>:"NT Read String Array.vi"("Name"="TestMode/TestList") -> ("String Array"=w616:string[])  [unwired: 9 in, 1 out]
        n317 = Build Array (concatenate)("Select the test to run...", w616) -> (w615:string[])
        n318 = property on="Test Name" class="Ring (strict)"("Strings []"=w615) -> ()  [unwired: 2 in, 2 out]
      }
      event "Test Name": Value Change {
        w618 = FALSE ("Visible")
        # "Tell the robot the test name to run"
        n319 = event-data() -> ("NewVal"=w622:u16)  [unwired: 1 in]
        n320 = property on="Test Name" class="Ring (strict)"() -> ("Strings []"=w623:string[])  [unwired: 2 in, 2 out]
        n321 = local write "Progress"(T18 {"Test Progress"=0, "Test Progress Text"=""} ("Progress")) -> ()
        n322 = Index Array(array=w623, index=w622) -> (element=w621:string)
        n323 = call <vilib>:"NT Write String.vi"("String"=w621, "Name"="TestMode/TestName") -> ()  [unwired: 9 in, 1 out]
        n324 = property on="Progress" class="Clust (strict)"("Visible"=TRUE) -> ()  [unwired: 2 in, 2 out]
        n325 = property on="Motor" class="Clust (strict)"("Visible"=w618) -> ()  [unwired: 2 in, 2 out]
        n326 = property on="Test Slider" class="Slide (strict)"("Visible"=w618) -> ()  [unwired: 2 in, 2 out]
        n327 = property on="On/Off" class="Bool (strict)"("Visible"=w618) -> ()  [unwired: 2 in, 2 out]
        n328 = property on="Rev/Fwd" class="Clust (strict)"("Visible"=w618) -> ()  [unwired: 2 in, 2 out]
        n329 = property on="Test Ring" class="Ring (strict)"("Visible"=w618) -> ()  [unwired: 2 in, 2 out]
      }
      event "Listbox": Double Click {
        n330 = event-data() -> ("PlatMods.Shift"=w626:bool, "Row"=w628:i32)  [unwired: 1 in]
        n331 = case shown="True" w626 {
          tunnel: w628 -> [w632 _]
          tunnel: 1 -> [w631 _]
          frame False {
            n332 = property on="Listbox" class="LstBox (strict)"() -> ("Item Symbols"=w630:i32[])  [unwired: 2 in, 2 out]
            n333 = Replace Array Subset(array=w630, new element=w631, index=w632) -> (w629:i32[])
            n334 = property on="Listbox" class="LstBox (strict)"("Item Symbols"=w629) -> ()  [unwired: 2 in, 2 out]
          }
          frame True {
            w633 = 0 ("Top Row")
            n335 = property on="Listbox" class="LstBox (strict)"() -> ("Number of Rows"=w635:u32)  [unwired: 2 in, 2 out]
            n336 = Initialize Array(0, w635) -> (w634:i32[])
            n337 = property on="Listbox" class="LstBox (strict)"("Top Row"=w633, "Value"=w633, "Item Symbols"=w634) -> ()  [unwired: 2 in, 2 out]
          }
        }
      }
      event "Listbox": Key Down {
        n338 = event-data() -> ("VKey"=w639:T32)  [unwired: 1 in]
        n339 = case shown="\"Left\", \"Right\"" w639 {
          selector: w639 -> [w644 _]
          tunnel: eventvkey."Left" ("VKey") -> [w642 _]
          frame "Left", "Right" {
            n340 = Equal?(x=w642, y=w644) -> (x = y?=w643:bool)
            n341 = Select(t=0, s=w643, f=1) -> (s? t:f=w645:i32)
            n342 = property on="Listbox" class="LstBox (strict)"() -> ("Item Symbols"=w648:i32[])  [unwired: 2 in, 2 out]
            n343 = Replace Array Subset(array=w648, new element=w645, index="Listbox") -> (w647:i32[])
            n344 = property on="Listbox" class="LstBox (strict)"("Item Symbols"=w647) -> ()  [unwired: 2 in, 2 out]
          }
          frame Default {
          }
        }
      }
      event "DB Camera Config": Value Change {
        n345 = event-data() -> ("NewVal"=w652:bool)  [unwired: 1 in]
        n346 = case shown="False" w652 {
          tunnel: w651 -> [w661 _]
          tunnel: [w654 w672] -> w650
          tunnel: w649 -> [w653 w672]
          frame False {
            w668 = "Camera"
            w671 = FALSE ("Visible")
            n347 = local read "Camera Settings"() -> (w660:T7)
            n348 = Index Array(array=w661) -> (element=w664:cluster{string[]})  [unwired: 1 in]
            n349 = Unbundle(w660) -> ("Frame Rate"=w659:i32, "Compression"=w658:i32, "Size"=w662:u16)
            n350 = Unbundle(w664) -> (w663:string[])
            n351 = Index Array(array=w663, index=w662) -> (element=w657:string)
            n352 = call-poly <vilib>:"Write Key.vi"("section"=w668, "value"=w657, "key"="Size", "refnum"=w653) -> ("refnum out"=w670:T24)  [unwired: 2 in, 5 out]
            n353 = call-poly <vilib>:"Write Key.vi"("section"=w668, "value"=w659, "key"="FrameRate", "refnum"=w670) -> ("refnum out"=w669:T24)  [unwired: 1 in, 6 out]
            n354 = property on="Camera Settings" class="Clust (strict)"("Visible"=w671) -> ()  [unwired: 2 in, 2 out]
            n355 = local write "DB Camera Config"(w671) -> ()
            n356 = call-poly <vilib>:"Write Key.vi"("section"=w668, "value"=w658, "key"="Compression", "refnum"=w669) -> ("refnum out"=w655:T24)  [unwired: 1 in, 6 out]
            n357 = call <vilib>:"Close Config Data.vi"("refnum"=w655) -> ("file path"=w656:path)  [unwired: 2 in, 8 out]
            n358 = call <vilib>:"Open Config Data.vi"("configuration file path"=w656) -> ("refnum"=w654:T24)  [unwired: 8 in, 2 out]
          }
          frame True {
            n359 = property on="Camera Settings" class="Clust (strict)"("Visible"=TRUE) -> ()  [unwired: 2 in, 2 out]
          }
        }
      }
      event "Camera Settings": Value Change {
        n360 = event-data() -> ("NewVal"=w685:T7)  [unwired: 1 in]
        n361 = Index Array(array=w681) -> (element=w680:cluster{string[]})  [unwired: 1 in]
        n362 = Unbundle(w685) -> ("Frame Rate"=w676:i32, "Compression"=w675:i32, "Size"=w678:u16)
        n363 = Unbundle(w680) -> (w679:string[])
        n364 = Index Array(array=w679, index=w678) -> (element=w677:string)
        n365 = Format Into String(format string="%s   %dfps   %d%%", w677, w676, w675) -> (resulting string=w682:string)  [unwired: 2 in, 1 out]
        n366 = Build Array(w682) -> (w683:string[])
        n367 = property on="DB Camera Config" class="Bool (strict)"("Strings [4]"=w683) -> ()  [unwired: 2 in, 2 out]
      }
      event "Motor.Enable": Value Change {
        n368 = event-data() -> ("NewVal"=w691:bool)  [unwired: 1 in]
        n369 = Unbundle("Motor") -> ("Value"=w690:dbl)  [unwired: 1 out]
        n370 = Select(t=w690, s=w691, f=0.0) -> (s? t:f=w688:dbl)
        n371 = call <vilib>:"NT Write Number.vi"("Numeric"=w688, "Name"=w687) -> ()  [unwired: 9 in, 1 out]
      }
      event "Test Slider": Value Change {
        n372 = event-data() -> ("NewVal"=w694:dbl)  [unwired: 1 in]
        n373 = call <vilib>:"NT Write Number.vi"("Numeric"=w694, "Name"=w695) -> ()  [unwired: 9 in, 1 out]
      }
      event "On/Off": Value Change {
        n374 = event-data() -> ("NewVal"=w699:bool)  [unwired: 1 in]
        n375 = Boolean To (0,1)(Boolean=w699) -> (0, 1=w698:i16)
        n376 = call <vilib>:"NT Write Number.vi"("Numeric"=w698, "Name"=w697) -> ()  [unwired: 9 in, 1 out]
      }
      event "Rev/Fwd": Value Change {
        n377 = event-data() -> ("NewVal.Forward"=w707:bool, "NewVal.Reverse"=w706:bool)  [unwired: 1 in]
        n378 = Boolean To (0,1)(Boolean=w707) -> (0, 1=w703:i16)
        n379 = Boolean To (0,1)(Boolean=w706) -> (0, 1=w705:i16)
        n380 = Negate(x=w705) -> (-x=w704:i16)
        n381 = Add(x=w703, y=w704) -> (x+y=w702:i16)
        n382 = call <vilib>:"NT Write Number.vi"("Numeric"=w702, "Name"=w701) -> ()  [unwired: 9 in, 1 out]
      }
      event "Test Ring": Value Change {
        n383 = event-data() -> ("NewVal"=w711:u16)  [unwired: 1 in]
        n384 = property on="Test Ring" class="Ring (strict)"() -> ("Strings []"=w712:string[])  [unwired: 2 in, 2 out]
        n385 = Index Array(array=w712, index=w711) -> (element=w710:string)
        n386 = call <vilib>:"NT Write String.vi"("String"=w710, "Name"=w709) -> ()  [unwired: 9 in, 1 out]
      }
      event "Rec Mode": Value Change {
        # "Update globals for recording mode and path to read log from.\nClear when logging and let NetworkTables set path for vision to\nuse."
        n387 = event-data() -> ("NewVal"=w722:enum32{"Stop", "Record", "Playback"})  [unwired: 1 in]
        n388 = global write "WPI_DashboardLogging Global.vi" "Logging Filename"(path "") -> ()
        n389 = case shown="\"Stop\", \"Record\"" w722 {
          tunnel: w721 -> [_ w724 w732]
          tunnel: [_ _ w731] -> w718
          tunnel: [_ _ w730] -> _
          tunnel: w716 -> [_ _ w728]
          tunnel: cluster{i32, i32} {-250, 170} -> [_ _ w727]
          tunnel: [_ _ T33 {"Image Size"=TRUE, "Image Type"=TRUE, "Pixel Value"=TRUE, "ROI Information"=TRUE, "Zoom Factor"=FALSE} ("Image Information Shown:All Elements")] -> w714
          tunnel: [_ _ TRUE ("Zoom Factor")] -> w713
          frame Default {
          }
          frame "Stop", "Record" {
            # "Place Window too"
            n390 = invoke class="VI" method="FP.Close"(reference=w724) -> (reference out=w723:refnum<vi>)  [unwired: 2 in, 2 out]
            n391 = invoke class="VI" method="Abort VI"(reference=w723) -> ()  [unwired: 2 in, 3 out]
          }
          frame "Playback" {
            n392 = call "Open Playback Panel.vi"("Offset"=w727, "DB VI Ref"=w728, "Playback in"=w732) -> ("Playback out"=w729:refnum<vi>)  [unwired: 8 in]
            n393 = register-events(w729) -> (reference out=w731:refnum<event-registration>, error out=w730:errorcluster)  [unwired: 2 in]
          }
        }
        n394 = global write "WPI_DashboardLogging Global.vi" "Recording"(w722) -> ()
        n395 = property on="Camera Image" class="ImageControl"("Image Information Shown"=w714, "Image Information Visible"=w713) -> ()  [unwired: 2 in, 2 out]
        n396 = call <vilib>:"WPI_DashboardNT Log FieldName Cache.vi"("Operation"=enum16{"Lookup/Add", "Index", "Clear"}."Clear") -> ()  [unwired: 8 in, 3 out]
      }
      event Panel Close {
        w733 = enum32{"Stop", "Record", "Playback"}."Stop" ("Rec Mode")
        n397 = event-data() -> ()  [unwired: 1 in, 4 out]
        n398 = local write "Rec Mode"(w733) -> ()
        n399 = global write "WPI_DashboardLogging Global.vi" "Recording"(w733) -> ()
      }
      event Panel Close {
        # "Abort playback window and ourself"
        n400 = event-data() -> ()  [unwired: 1 in, 4 out]
        n401 = invoke class="VI" method="FP.Close"(reference=w738) -> (reference out=w737:refnum<vi>)  [unwired: 2 in, 2 out]
        n402 = invoke class="VI" method="Abort VI"(reference=w737) -> (error out=w736:errorcluster)  [unwired: 2 in, 2 out]
        n403 = invoke class="VI" method="Abort VI"(error in=w736) -> ()  [unwired: 2 in, 3 out]
      }
    }
  }
  n404 = property on="On/Off" class="Bool (strict)"("Visible"=w49) -> ()  [unwired: 2 in, 2 out]
  n405 = property on="Motor" class="Clust (strict)"("Visible"=w49) -> ()  [unwired: 2 in, 2 out]
  n406 = property on="Progress" class="Clust (strict)"("Visible"=w49) -> ()  [unwired: 2 in, 2 out]
  n407 = property on="Test Ring" class="Ring (strict)"("Visible"=w49) -> ()  [unwired: 2 in, 2 out]
  n408 = property on="Rev/Fwd" class="Clust (strict)"("Visible"=w49) -> ()  [unwired: 2 in, 2 out]
  n409 = property on="Camera Settings" class="Clust (strict)"("Visible"=w49) -> ()  [unwired: 2 in, 2 out]
  n410 = local write "DB Camera Config"(w49) -> ()
  n411 = global write "WPI_DashboardLogging Global.vi" "Recording"(w32) -> ()
  n412 = local write "Rec Mode"(w32) -> ()
  n413 = call <vilib>:"Sound Input Stop.vi"("error in (no error)"=w17, "task ID"=w16) -> ("error out"=w15:errorcluster, "task ID out"=w14:T25)  [unwired: 8 in]
  n414 = call <vilib>:"Sound Input Clear.vi"("error in (no error)"=w15, "task ID"=w14) -> ()  [unwired: 9 in, 1 out]
